vi "getIsReferenced.vi"(8 "error in (no error)":errorcluster, 11 "IProperty in":refnum<class "IProperty.lvclass">) -> (0 "error out":errorcluster, 2 "IsReferenced?":bool, 3 "IProperty out":refnum<class "IProperty.lvclass">)   [LabVIEW 2022 SP3, in "openDAQ.lvlib" / "IBaseObject.lvlib" / "IProperty.lvlib" / "IProperty.lvclass"]
uses:
  <instrlib>/openDAQ/Public/Classes/IProperty/IProperty.lvclass
  <instrlib>/openDAQ/Public/Classes/IProperty/IProperty.lvclass/IProperty.ctl
  <instrlib>/openDAQ/Binaries/Windows/x86/copendaq32.dll
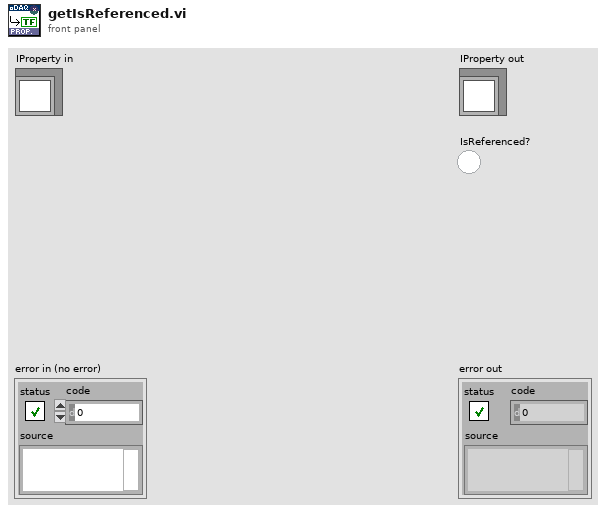
[diagram p1: front panel]
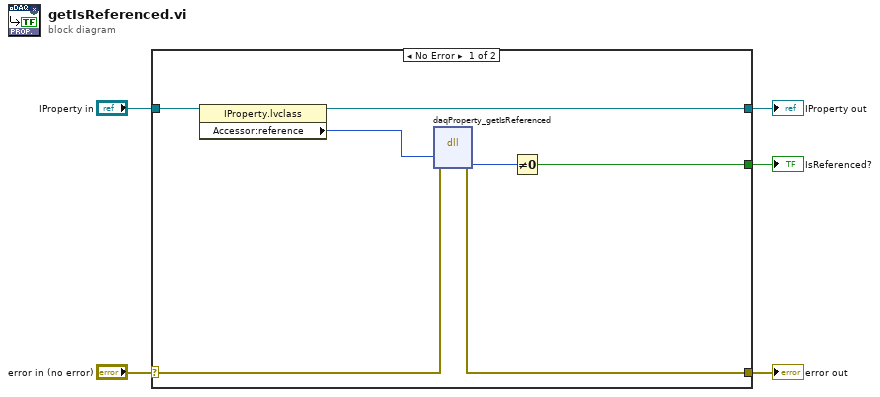
[diagram p0: block diagram]
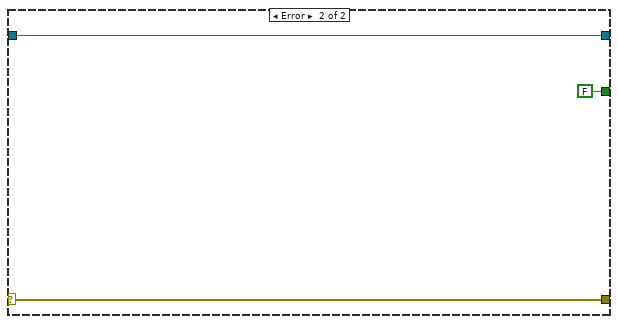
[diagram p2: hidden frame]
diagram:
  n1 = case shown="No Error" "error in (no error)" {
    selector: "error in (no error)" -> [w6 w15]
    tunnel: [w7 w15] -> w4
    tunnel: [w11 w14] -> w2
    tunnel: "IProperty in" -> [w12 w14]
    tunnel: [w8 FALSE] -> w1
    frame No Error {
      n2 = property class="IProperty.lvclass"(reference=w12) -> (reference out=w11:refnum<class "IProperty.lvclass">, "Accessor:reference"=w10:i64)  [unwired: 1 in, 1 out]
      n3 = dll-call lib="C:/Program Files (x86)/National Instruments/LabVIEW 2022/instr.lib/openDAQ/Binaries/Windows/x86/copendaq*.*" fn="daqProperty_getIsReferenced"(error in=w6, "property"=w10) -> (error out=w7:errorcluster, "isReferenced"=w9:i64)  [unwired: 5 in, 1 out]
      n4 = Not Equal To 0?(x=w9) -> (x != 0?=w8:bool)
    }
    frame Error {
    }
  }
  "error out" <- w4
  "IProperty out" <- w2
  "IsReferenced?" <- w1
